vi "remove_content_in_[].vi"(8 "error in (no error)":errorcluster, 11 "Instrument Command In":string) -> (0 "error out":errorcluster, 3 "Instrument Command Out":string)   [LabVIEW 2018]
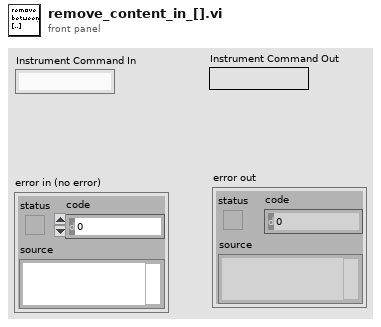
[diagram p1: front panel]
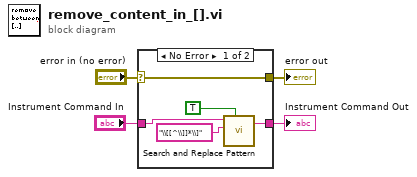
[diagram p0: block diagram]
diagram:
  n1 = case shown="No Error" "error in (no error)" {
    selector: "error in (no error)" -> [w5 w10]
    tunnel: "Instrument Command In" -> [w8 w11]
    tunnel: [w7 w11] -> w3
    tunnel: [w5 w10] -> w1
    frame No Error {
      n2 = call <vilib>:"Search and Replace Pattern.vi"("string"=w8, "regular expression (\"\")"="\\[[^\\]]*\\]" ("regular expression (\"\")"), "replace all? (F)"=TRUE) -> ("result string"=w7:string)  [unwired: 1 in, 2 out]
    }
    frame Error {
    }
  }
  "Instrument Command Out" <- w3
  "error out" <- w1
